vi "Update Channels.vi"(8 "error in":errorcluster, 9 "Analog":bool, 10 "Previous Number of Channels":i32=8, 11 "Plugin in":refnum<class "Sequencer with Output Values.lvclass">) -> (0 "error out":errorcluster, 2 "Updated Number of Channels":i32, 3 "Plugin out":refnum<class "Sequencer with Output Values.lvclass">)   [LabVIEW 2020, in "Sequencer with Output Values.lvlib" / "Sequencer with Output Values.lvclass"]
uses:
  Sequencer with Output Values.lvclass
  C:/Program Files/National Instruments/LabVIEW 2024/vi.lib/FlexLogger/SDK/PluginSDK.lvlibp/PEFClasses/SDK/Plugin/Plugin.lvclass
  <vilib>/FlexLogger/SDK/PluginSDK.lvlibp/PEFClasses/SDK/Channel/Data Type.ctl
  <vilib>/FlexLogger/SDK/PluginSDK.lvlibp/PEFClasses/SDK/Producer Channel/Producer Channel.lvclass
  C:/Program Files/National Instruments/LabVIEW 2024/vi.lib/FlexLogger/SDK/PluginSDK.lvlibp/PEFClasses/SDK/Channel/Channel.lvclass
  Global Strings.vi
  <vilib>/FlexLogger/SDK/PluginSDK.lvlibp/PEFClasses/SDK/Plugin/ParameterAccess/Read I32.vi
  <vilib>/FlexLogger/SDK/PluginSDK.lvlibp/PEFClasses/SDK/Plugin/ParameterAccess/Write I32.vi
  <vilib>/FlexLogger/SDK/PluginSDK.lvlibp/PEFClasses/SDK/Producer Channel/Create Producer Channel.vi
  <vilib>/FlexLogger/SDK/PluginSDK.lvlibp/PEFClasses/SDK/Plugin/Plugin.lvclass
  <vilib>/FlexLogger/SDK/PluginSDK.lvlibp
  C:/Program Files/National Instruments/LabVIEW 2024/vi.lib/FlexLogger/SDK/PluginSDK.lvlibp/PEFClasses/SDK/Processing Element/Processing Element.lvclass
  C:/dev/niflexlogger-plugins/plugins/Sequencer with Output Values/source/Sequencer with Output Values/Sequencer with Output Values.lvclass
  <vilib>/FlexLogger/SDK/PluginSDK.lvlibp/PEFClasses/SDK/Channel/Channel.lvclass
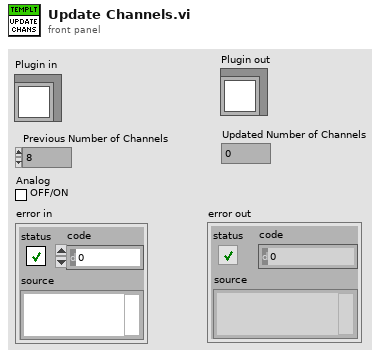
[diagram p1: front panel]
types:
  T1 = typedef "PluginSDK.lvlibp/Channel.lvclass/Data Type.ctl" = enum16{"Wfm (DBL)", "Wfm (Digital)"}
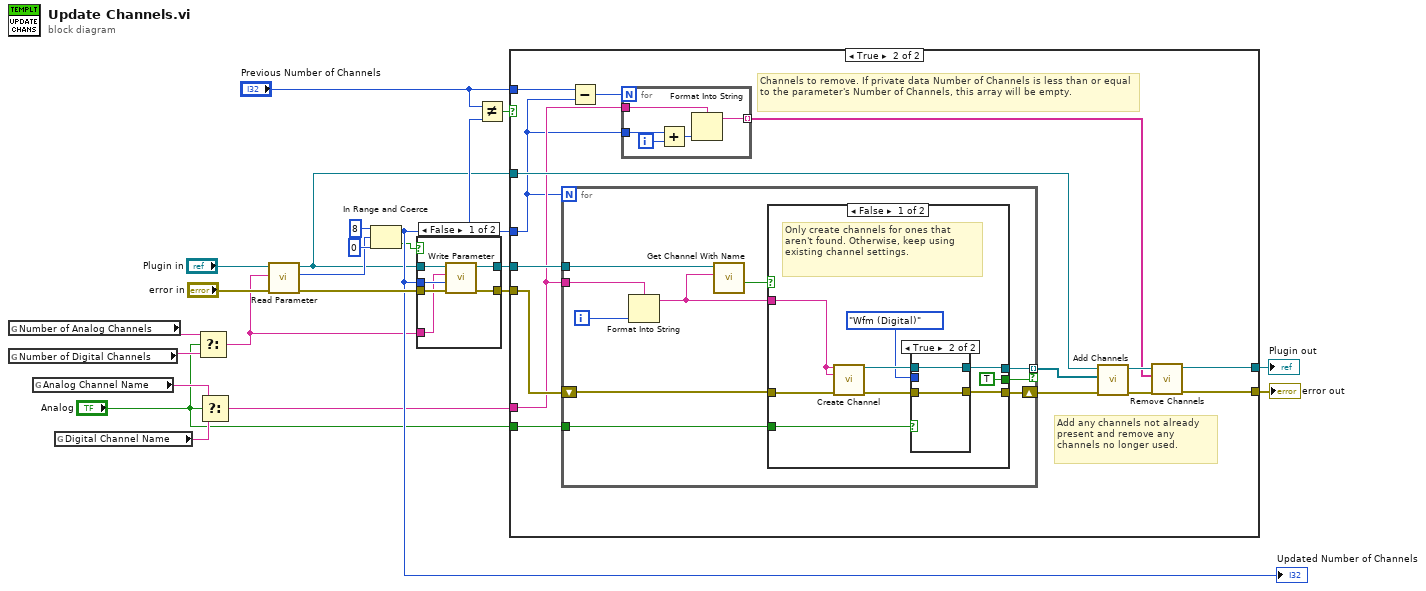
[diagram p0: block diagram]
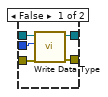
[diagram p4: hidden frame]
diagram:
  n1 = global read "Global Strings.vi" "Number of Analog Channels"() -> (w9:string)
  n2 = global read "Global Strings.vi" "Number of Digital Channels"() -> (w8:string)
  n3 = global read "Global Strings.vi" "Analog Channel Name"() -> (w6:string)
  n4 = global read "Global Strings.vi" "Digital Channel Name"() -> (w5:string)
  n5 = Select(t=w9, s="Analog", f=w8) -> (s? t:f=w7:string)
  n6 = Select(t=w6, s="Analog", f=w5) -> (s? t:f=w4:string)
  n7 = call-poly <vilib>:"Read Parameter.vi"("error in (no error)"="error in", "Name"=w7, "Plugin in"="Plugin in") -> ("error out"=w19:errorcluster, "Value"=w18:i32, "Plugin out"=w13:refnum<class "Sequencer with Output Values.lvclass">)  [unwired: 5 in, 1 out]
  n8 = In Range and Coerce(upper limit=8, x=w18, lower limit=0) -> (coerced(x)=w17:i32, In Range?=w16:bool)
  "Updated Number of Channels" <- w17
  n9 = case shown="False" w16 {
    tunnel: w13 -> [w28 w30]
    tunnel: w19 -> [w27 w29]
    tunnel: w17 -> [w26 _]
    tunnel: w7 -> [w25 _]
    tunnel: [w24 w30] -> w15
    tunnel: [w23 w29] -> w14
    frame False {
      n10 = call-poly <vilib>:"Write Parameter.vi"("error in (no error)"=w27, "Value"=w26, "Name"=w25, "Plugin in"=w28) -> ("error out"=w23:errorcluster, "Plugin out"=w24:refnum<class "Sequencer with Output Values.lvclass">)  [unwired: 6 in]
    }
    frame True {
    }
  }
  n11 = Not Equal?(x="Previous Number of Channels", y=w17) -> (x != y?=w22:bool)
  n12 = case shown="True" w22 {
    tunnel: "Previous Number of Channels" -> [_ w47]
    tunnel: w17 -> [_ w33]
    tunnel: w15 -> [w32 w45]
    tunnel: w14 -> [w31 w44]
    tunnel: w13 -> [_ w36]
    tunnel: [w32 w38] -> w3
    tunnel: [w31 w37] -> w2
    tunnel: w4 -> [_ w35]
    tunnel: "Analog" -> [_ w34]
    frame False {
    }
    frame True {
      # "Add any channels not already present and remove any channels no longer used."
      # "Channels to remove. If private data Number of Channels is less than or equal to the parameter's Number of Channels, this array will be empty."
      n13 = for {
        N: w33 -> [_]
        tunnel: w45 -> [w57]
        tunnel: [w54] -> w42 mode=indexing if=w53
        shift-right: [w52] -> w43
        shift-left: w44 -> [w51]
        tunnel: w35 -> [w50]
        tunnel: w34 -> [w49]
        i -> [w48]
        n14 = Format Into String(format string=w50, w48) -> (resulting string=w55:string)  [unwired: 2 in, 1 out]
        n15 = call <vilib>:"Get Channel With Name.vi"("Name"=w55, "Plugin in"=w57) -> ("Found?"=w56:bool)  [unwired: 7 in, 2 out]
        n16 = case shown="False" w56 {
          tunnel: w55 -> [w64 _]
          tunnel: [w59 _] -> w54
          tunnel: [TRUE _] -> w53
          tunnel: [w58 w74] -> w52
          tunnel: w51 -> [w65 w74]
          tunnel: w49 -> [w63 _]
          frame False {
            # "Only create channels for ones that aren't found. Otherwise, keep using existing channel settings."
            n17 = call-poly <vilib>:"Create Channel.vi"("Unique Channel Identifier"=w64, "Default Channel Name"=w64, "error in (no error)"=w65) -> ("Producer Channel"=w62:refnum<class "Producer Channel.lvclass">, "error out"=w60:errorcluster)  [unwired: 11 in]
            n18 = case shown="True" w63 {
              tunnel: w62 -> [w71 w73]
              tunnel: Data_Type."Wfm (Digital)" ("Data Type") -> [w70 _]
              tunnel: w60 -> [w69 w72]
              tunnel: [w68 w73] -> w59
              tunnel: [w67 w72] -> w58
              frame False {
                n19 = call-dynamic "Write Data Type.vi"("error in (no error)"=w69, "Data Type"=w70, "Channel in"=w71) -> ("error out"=w67:errorcluster, "Channel out"=w68:refnum<class "Producer Channel.lvclass">)  [unwired: 7 in]
              }
              frame True {
              }
            }
          }
          frame True {
          }
        }
      }
      n20 = Subtract(x=w47, y=w33) -> (x-y=w46:i32)
      n21 = for {
        N: w46 -> [_]
        tunnel: [w79] -> w39 mode=indexing
        tunnel: w33 -> [w77]
        tunnel: w35 -> [w75]
        i -> [w78]
        n22 = Add(x=w77, y=w78) -> (x+y=w76:i32)
        n23 = Format Into String(format string=w75, w76) -> (resulting string=w79:string)  [unwired: 2 in, 1 out]
      }
      n24 = call <vilib>:"Add Channels.vi"("error in (no error)"=w43, "Channels"=w42, "Plugin in"=w36) -> ("error out"=w41:errorcluster, "Plugin out"=w40:refnum<class "Sequencer with Output Values.lvclass">)  [unwired: 7 in]
      n25 = call-dynamic "Remove Channels.vi"("error in (no error)"=w41, "Unique Channel Identifiers to Delete"=w39, "Plugin in"=w40) -> ("error out"=w37:errorcluster, "Plugin out"=w38:refnum<class "Sequencer with Output Values.lvclass">)  [unwired: 7 in]
    }
  }
  "Plugin out" <- w3
  "error out" <- w2
